vi "exposureTimeGet.vi"(2 "exposureUnitsPrefix":dbl=1000000.0, 4 "error in":errorcluster, 5 "Session in":T1) -> (0 "errorOut":errorcluster, 1 "exposureTime":dbl)   [LabVIEW 2021]
uses:
  <vilib>/userdefined/High Color/IMAQdx.ctl
  <resource>/objmgr/imaqdx.rc
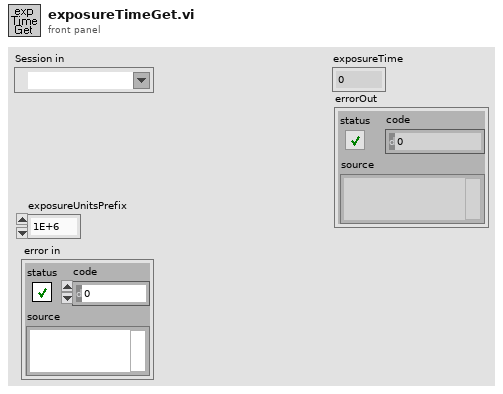
[diagram p1: front panel]
types:
  T1 = typedef "IMAQdx.ctl" = refnum<k21>
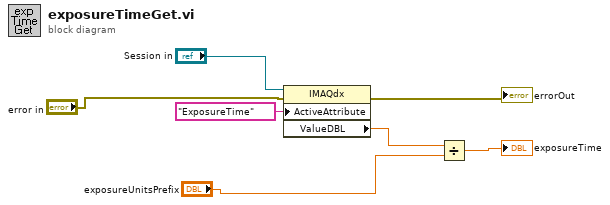
[diagram p0: block diagram]
diagram:
  n1 = property class="IMAQdx"(reference="Session in", error in="error in", "ActiveAttribute"="ExposureTime") -> (error out=→"errorOut":errorcluster, "ValueDBL"=w6:dbl)  [unwired: 1 out]
  n2 = Divide(x=w6, y="exposureUnitsPrefix") -> (x/y=→"exposureTime":dbl)
